vi "Change Position.vi"(8 "error in (no error)":errorcluster, 10 "Change Position":i16, 11 "SwipeMenu in":refnum<class "SwipeMenu.lvclass">) -> (0 "error out":errorcluster, 2 "In Range?":bool, 3 "SwipeMenu out":refnum<class "SwipeMenu.lvclass">)   [LabVIEW 2019, in "SwipeMenu.lvclass"]
uses:
  SwipeMenu.lvclass
  SwipeMenu.lvclass/SwipeMenu.ctl
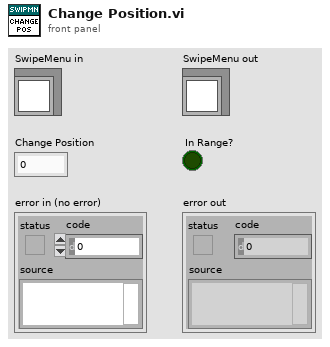
[diagram p1: front panel]
types:
  T1 = enum8{"Enabled", "Disabled", "Disabled and Grayed Out"}
  T2 = typedef "LVRectTypeDef.ctl" = cluster{"Left":i16, "Top":i16, "Right":i16, "Bottom":i16}
  T3 = typedef "LVPointTypeDef.ctl" = cluster{"Horizontal":i16, "Vertical":i16}
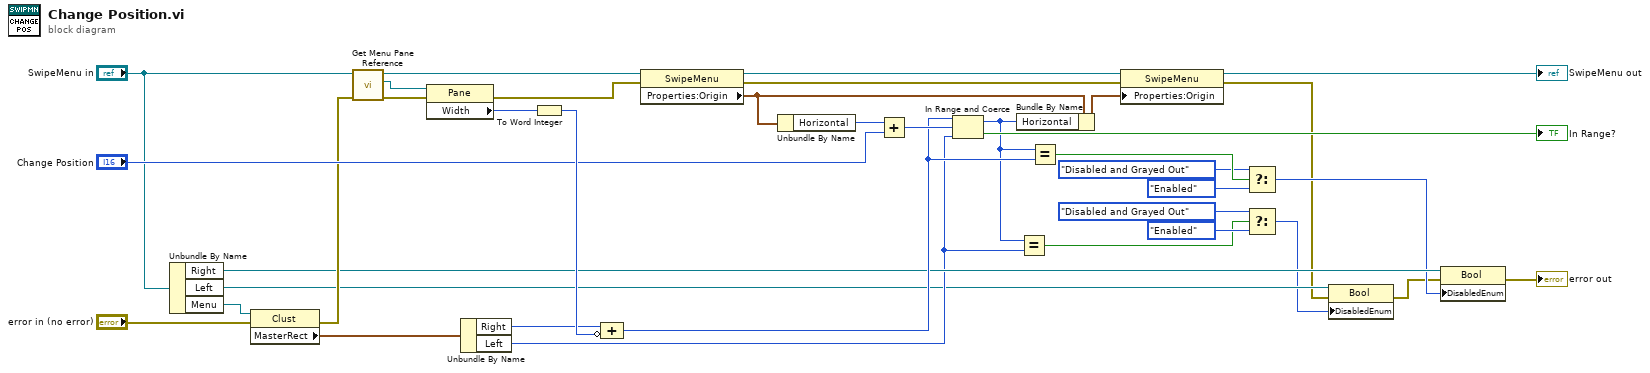
[diagram p0: block diagram]
diagram:
  n1 = Unbundle By Name("SwipeMenu in") -> ("Right"=w14:refnum<vi>, "Left"=w5:refnum<vi>, "Menu"=w37:refnum<vi>)
  n2 = property class="Clust"(reference=w37, error in="error in (no error)") -> (error out=w19:errorcluster, "MasterRect"=w33:T2)  [unwired: 1 out]
  n3 = call "Get Menu Pane Reference.vi"("error in (no error)"=w19, "SwipeMenu in"="SwipeMenu in") -> ("error out"=w20:errorcluster, "Menu Pane Refnum"=w23:refnum<vi>, "SwipeMenu out"=w22:refnum<class "SwipeMenu.lvclass">)  [unwired: 7 in]
  n4 = property class="Pane"(reference=w23, error in=w20) -> (error out=w21:errorcluster, "Width"=w35:u32)  [unwired: 1 out]
  n5 = Unbundle By Name(w33) -> ("Right"=w34:i16, "Left"=w9:i16)
  n6 = To Word Integer(number=w35) -> (16bit integer=w36:i16)
  n7 = Compound Arithmetic op=ADD(w34, invert w36) -> (w16:i16)
  n8 = property class="SwipeMenu"(reference=w22, error in=w21) -> (reference out=w27:refnum<class "SwipeMenu.lvclass">, error out=w30:errorcluster, "Properties:Origin"=w28:T3)
  n9 = Unbundle By Name(w28) -> ("Horizontal"=w31:i16)
  n10 = Add(x=w31, y="Change Position") -> (x+y=w25:i16)
  n11 = In Range and Coerce(upper limit=w16, x=w25, lower limit=w9) -> (coerced(x)=w10:i16, In Range?=→"In Range?":bool)
  n12 = Bundle By Name(cluster=w28, "Horizontal"=w10) -> (w29:T3)
  n13 = Equal?(x=w10, y=w9) -> (x = y?=w6:bool)
  n14 = Equal?(x=w10, y=w16) -> (x = y?=w15:bool)
  n15 = property class="SwipeMenu"(reference=w27, error in=w30, "Properties:Origin"=w29) -> (reference out=→"SwipeMenu out":refnum<class "SwipeMenu.lvclass">, error out=w2:errorcluster)
  n16 = Select(t=T1."Disabled and Grayed Out" ("Disabled"), s=w15, f=T1."Enabled" ("Disabled")) -> (s? t:f=w11:T1)
  n17 = Select(t=T1."Disabled and Grayed Out" ("Disabled"), s=w6, f=T1."Enabled" ("Disabled")) -> (s? t:f=w4:T1)
  n18 = property class="Bool"(reference=w5, error in=w2, "DisabledEnum"=w4) -> (error out=w3:errorcluster)  [unwired: 1 out]
  n19 = property class="Bool"(reference=w14, error in=w3, "DisabledEnum"=w11) -> (error out=→"error out":errorcluster)  [unwired: 1 out]
